vi "Import Custom Device.vi"   [LabVIEW 2020, in "Ballard MIL-STD-1553 Scripting.lvlib"]
uses:
  Ballard MIL-STD-1553 Scripting.lvlib
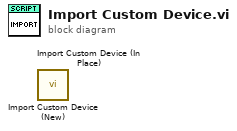
[diagram p0: block diagram]
diagram:
  n1 = call "Import Custom Device (New).vi"() -> ()  [unwired: 9 in, 3 out]
  n2 = call "Import Custom Device (In Place).vi"() -> ()  [unwired: 10 in, 2 out]
